vi "Set Shooter PID.vi"(11 "Setpoint":dbl) -> ()   [LabVIEW 2015]
uses:
  <vilib>/addons/control/pid/pid.llb/PID (DBL).vi
  <vilib>/addons/control/pid/NI_PID_pid.lvlib
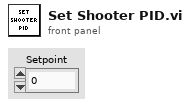
[diagram p1: front panel]
types:
  T1 = cluster{"proportional gain (Kc)":dbl, "integral time (Ti, min)":dbl, "derivative time (Td, min)":dbl}
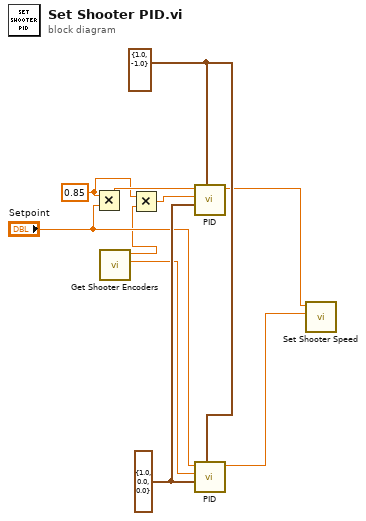
[diagram p0: block diagram]
diagram:
  w3 = 0.85 ("x")
  w8 = T1 {"proportional gain (Kc)"=1.0, "integral time (Ti, min)"=0.0, "derivative time (Td, min)"=0.0} ("PID gains")
  w10 = cluster{"output high":dbl, "output low":dbl} {"output high"=1.0, "output low"=-1.0} ("output range")
  n1 = Multiply(x=w3, y="Setpoint") -> (x*y=w4:dbl)
  n2 = call "Get Shooter Encoders.vi"() -> ("Rate Enc1"=w7:dbl, "Rate Enc2"=w1:dbl)  [unwired: 10 in]
  n3 = Multiply(x=w3, y=w1) -> (x*y=w2:dbl)
  n4 = call-poly <vilib>:"PID.vi"("output range"=w10, "PID gains"=w8, "process variable"=w2, "setpoint"=w4) -> ("output"=w6:dbl)  [unwired: 6 in, 1 out]
  n5 = call-poly <vilib>:"PID.vi"("output range"=w10, "PID gains"=w8, "process variable"=w7, "setpoint"="Setpoint") -> ("output"=w9:dbl)  [unwired: 6 in, 1 out]
  n6 = call "Set Shooter Speed.vi"("Set Bottom Speed"=w9, "Set Top Speed"=w6) -> ()  [unwired: 10 in]
